vi "test_alignRightWithValidation.vi"(11 "Test Case In":refnum<class "RelativeAlignmentTests.lvclass">) -> (0 "error out":errorcluster, 3 "Test Case Out":refnum<class "RelativeAlignmentTests.lvclass">)   [LabVIEW 2023, in "RelativeAlignmentTests.lvclass"]
uses:
  RelativeAlignmentTests.lvclass
  C:/Program Files (x86)/National Instruments/LabVIEW 2023/vi.lib/Astemes/LUnit/Test Case.lvclass
  <vilib>/Astemes/LUnit/Test Case.lvclass/Test Case.ctl
  <vilib>/Astemes/LUnit/Core/LUnit Test Case/Private/Append Fail Result.vi
  <vilib>/Astemes/LUnit/Core/LUnit Test Case/Private/Append Pass Result.vi
  <vilib>/Astemes/LUnit/Core/LUnit Test Case/Private/Run In UI.vi
  <vilib>/Utility/error.llb/Clear Errors.vi
  <vilib>/Astemes/LUnit/Test Case.lvclass
  source/TLC_Geometry.lvlib
panel:
  in  "movingObject":string
  in  "anchor":dbl
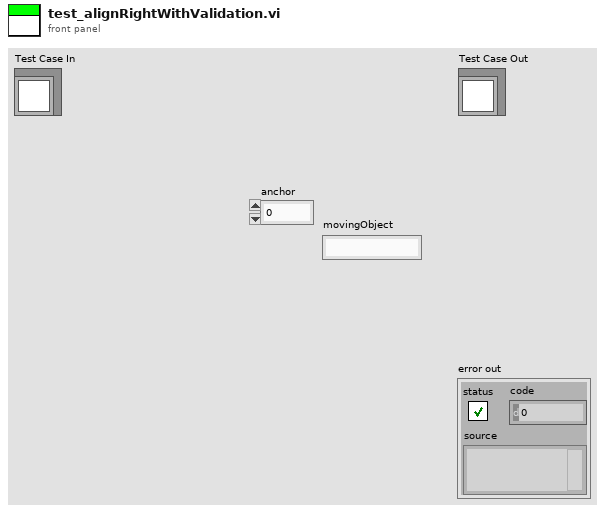
[diagram p1: front panel]
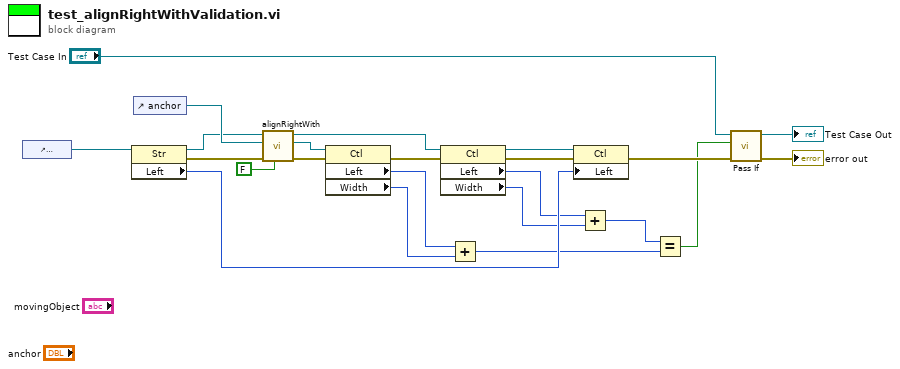
[diagram p0: block diagram]
diagram:
  n1 = control-ref of="movingObject"() -> (w14:refnum<vi>)
  n2 = property class="Str"(reference=w14) -> (reference out=w13:refnum<vi>, error out=w21:errorcluster, "Left"=w11:i32)  [unwired: 1 in]
  n3 = control-ref of="anchor"() -> (w22:refnum<vi>)
  n4 = call "alignRightWith.vi"("useControlBodyOnly"=FALSE, "error in (no error)"=w21, "anchorObject"=w22, "movingObject"=w13) -> ("error out"=w20:errorcluster, "anchorObject(dup)"=w18:refnum<vi>, "movingObject(dup)"=w17:refnum<vi>)  [unwired: 5 in]
  n5 = property class="Ctl"(reference=w18, error in=w20) -> (error out=w19:errorcluster, "Left"=w5:i32, "Width"=w6:u32)  [unwired: 1 out]
  n6 = property class="Ctl"(reference=w17, error in=w19) -> (reference out=w15:refnum<vi>, error out=w16:errorcluster, "Left"=w2:i32, "Width"=w3:u32)
  n7 = Add(x=w5, y=w6) -> (x+y=w4:u32)
  n8 = property class="Ctl"(reference=w15, error in=w16, "Left"=w11) -> (error out=w12:errorcluster)  [unwired: 1 out]
  n9 = Add(x=w2, y=w3) -> (x+y=w1:u32)
  n10 = Equal?(x=w1, y=w4) -> (x = y?=w10:bool)
  n11 = call <vilib>:"Pass If.vi"("error in (no error)"=w12, "Pass?"=w10, "LUnit Test Case In"="Test Case In") -> ("error out"=→"error out":errorcluster, "LUnit Test Case Out"=→"Test Case Out":refnum<class "RelativeAlignmentTests.lvclass">)  [unwired: 7 in]
